vi "Move and Delete Files.vi"(9 "target path":path, 10 "date/time string":string, 11 "source path":path) -> (3 "Write file":path)   [LabVIEW 2014]
uses:
  <vilib>/Utility/file.llb/Read From Spreadsheet File (string).vi
panel:
  out "string":string
  out "match substring":string
  out "before substring":string
  out "after substring":string
  out "concatenated string":string
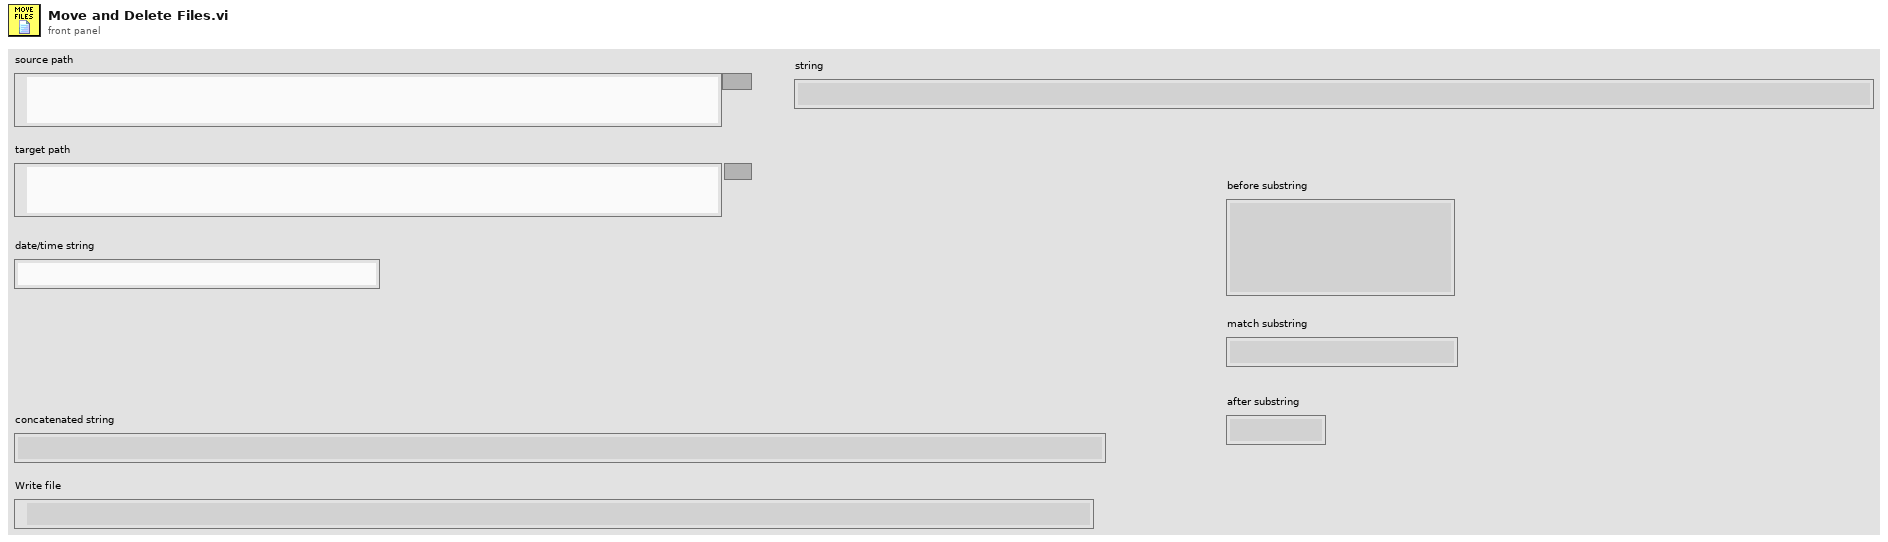
[diagram p1: front panel]
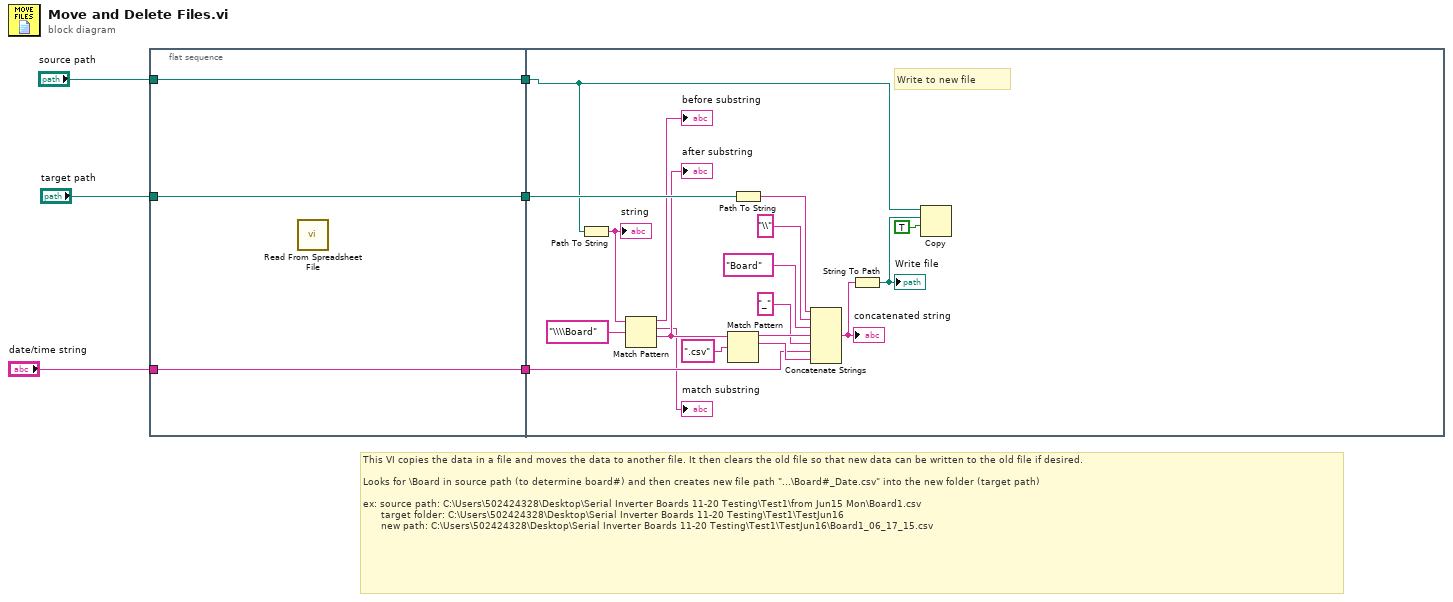
[diagram p0: block diagram]
diagram:
  # "This VI copies the data in a file and moves the data to another file. It then clears the old file so that new data can be written to the old file if desired.\n\nLooks for \\Board in source path (to determine board#) and then creates new file path \"...\\Board#_Date.csv\" into the new folder (target path)\n\nex: source path: C:\\Users\\502424328\\Desktop\\Serial Inverter Boards 11-20 Testing\\Test1\\from Jun15 Mon\\Board1.csv \n      target folder: C:\\Users\\502424328\\Desktop\\Serial Inverter Boards 11-20 Testing\\Test1\\TestJun16\n      new path: C:\\Users\\502424328\\Desktop\\Serial Inverter Boards 11-20 Testing\\Test1\\TestJun16\\Board1_06_17_15.csv"
  n1 = flat-sequence {
    tunnel: "source path" -> [w7]
    tunnel: "date/time string" -> [w8]
    tunnel: "target path" -> [w9]
    tunnel: [w9] -> w3
    tunnel: [w8] -> w2
    tunnel: [w7] -> w1
    tunnel: w3 -> [w24]
    tunnel: w2 -> [w16]
    tunnel: w1 -> [w22]
    frame #0 {
      n2 = call-poly <vilib>:"Read From Spreadsheet File.vi"() -> ()  [unwired: 7 in, 5 out]
    }
    frame #1 {
      # "Write to new file"
      n3 = Path To String(path=w22) -> (string=w10:string)
      "string" <- w10
      n4 = Match Pattern(string=w10, regular expression="\\\\Board") -> (before substring=→"before substring":string, match substring=→"match substring":string, after substring=w21:string)  [unwired: 1 in, 1 out]
      "after substring" <- w21
      n5 = Match Pattern(string=w21, regular expression=".csv") -> (before substring=w19:string, match substring=w17:string)  [unwired: 1 in, 2 out]
      n6 = Path To String(path=w24) -> (string=w23:string)
      n7 = Concatenate Strings(w23, "\\" ("string"), "Board" ("string"), w19, "_" ("string"), w16, w17) -> (w26:string)
      "concatenated string" <- w26
      n8 = String To Path(string=w26) -> (path=w25:path)
      "Write file" <- w25
      n9 = Copy(9:TRUE ("overwrite (F)"), 10:w25, 11:w22) -> ()  [unwired: 2 in, 3 out]
    }
  }
